vi "Unittest.vi"() -> ()   [LabVIEW 2017]
uses:
  Logger.lvclass
panel:
  out "String 2":string
  out "logs":string[][](array[string])
  in  "max logs":i64=100
  in  "String":string="abdc"
  in  "stop":bool
  in  "Add to log?":bool
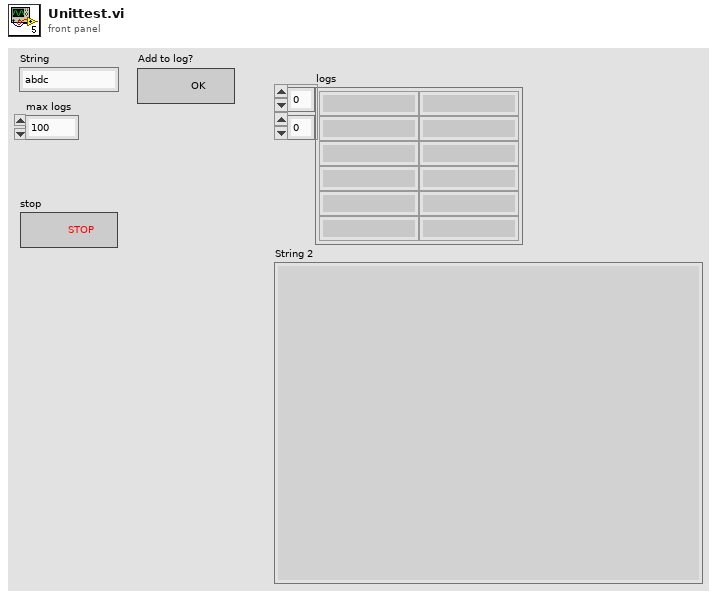
[diagram p1: front panel]
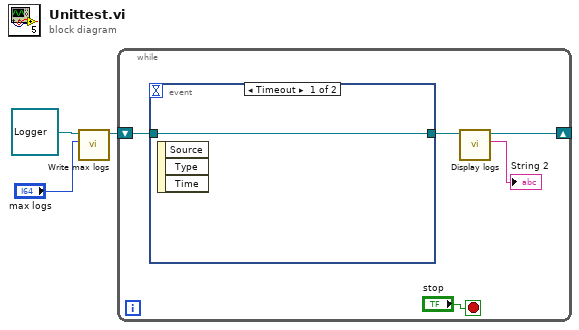
[diagram p0: block diagram]
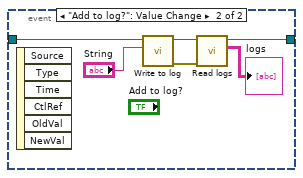
[diagram p2: hidden frame]
diagram:
  n1 = call-dynamic "Write max logs.vi"("max logs"="max logs", "Logger in"=refnum<class "Logger.lvclass"> refnum ("Logger.lvclass")) -> ("Logger out"=w2:refnum<class "Logger.lvclass">)  [unwired: 8 in, 1 out]
  n2 = while {
    shift-right: [w5] -> _
    shift-left: w2 -> [w8]
    stop <- "stop" stop-if-true
    n3 = event shown="[0] Timeout" {
      selector: _ -> [_ _]
      dyn-events: _ -> [_ _]
      timeout: _ -> [_ _]
      tunnel: w8 -> [w9 w12]
      tunnel: [w9 w11] -> w6
      event Timeout {
        n4 = event-data() -> ()  [unwired: 1 in, 3 out]
      }
      event "Add to log?": Value Change {
        n5 = event-data() -> ()  [unwired: 1 in, 6 out]
        n6 = call-dynamic "Write to log.vi"("Log"="String", "Logger in"=w12) -> ("error out"=w15:errorcluster, "Logger out"=w14:refnum<class "Logger.lvclass">)  [unwired: 8 in]
        n7 = call-dynamic "Read logs.vi"("error in (no error)"=w15, "Logger in"=w14) -> ("logs"=→"logs":string[][], "Logger out"=w11:refnum<class "Logger.lvclass">)  [unwired: 7 in, 1 out]
      }
    }
    n8 = call-dynamic "Display logs.vi"("Logger in"=w6) -> ("String"=→"String 2":string, "Logger out"=w5:refnum<class "Logger.lvclass">)  [unwired: 8 in, 1 out]
  }
